vi "Power Output Unflatten Test Parameters.vi"(9 "error in (no error)":errorcluster, 10 "Parameter String":string) -> (1 "error out":errorcluster, 2 "Power Verification Test Parameters":T2={"Stimulus"={"Frequency Type"=enum."Band Edges", "Frequency Ranges"=[], "TX 1 Frequency (MHz)"={"Min"=0.0, "Max"=0.0}, "TX 2 Frequency (MHz)"={"Min"=0.0, "Max"=0.0}, "RX Frequency (MHz)"={"Min"=0.0, "Max"=0.0}, "Pad Model Number"="", "Pad Serial Number"="", "Pad Values"=[]}, "Measurement"={"DUT Port"=enum."Port 1", "Direction"=0, "Frequency Step Size"=0}, "Display"={"Frequency"={"Min"=-1.0, "Max"=-1.0}, "Power"={"Min"=-1, "Max"=-1}}, "Limit"={"Min Power (dBm)"=44.0}, "Calibration"={"Calibrated?"=FALSE}} {"Measurement"."Frequency Step Size" items=["0.2", "0.4", "1.0", "2.0", "4.0"]; "Measurement"."Direction" items=["Reverse", "Forward", "Auxiliary"]}, 5 "Test Version":string)   [LabVIEW 2011]
uses:
  TypeDefs/Power Output Test Parameters.ctl
  TypeDefs/Power Output Stimulus Parameters.ctl
  TypeDefs/Power Output Measurement Parameters.ctl
  SI.LIB/PIM.LIB/HW IO/DUTport.ctl
  SI.LIB/PIM.LIB/HW IO/MeasMode.ctl
  SI.LIB/PIM.LIB/HW IO/PIM Sweep Step Size.ctl
  TypeDefs/Power Output Display Parameters.ctl
  TypeDefs/Power Output Limit Parameters.ctl
  TypeDefs/Power Output Calibration State.ctl
  Test Return Parameter.ctl
panel:
  in  "Return Parameter":T1
  out "Parameter Variant":variant
  in  "Required Instruments":string[](array[string])=["PIM", "PWM"]
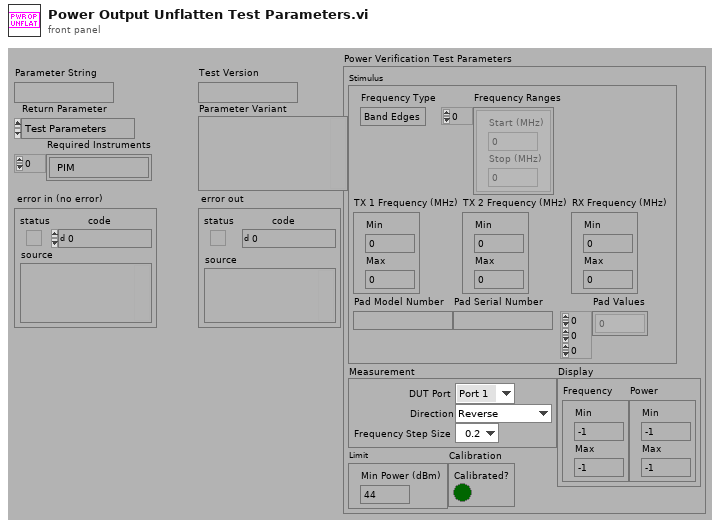
[diagram p1: front panel]
types:
  T1 = typedef "Test Return Parameter.ctl" = enum16{"Test Parameters", "Required Instruments", "Datasheets", "QuickMode"}
  T2 = typedef "Power Output Test Parameters.ctl" = cluster{"Stimulus":T3, "Measurement":T4, "Display":T8, "Limit":T9, "Calibration":T10}
  T3 = typedef "Power Output Stimulus Parameters.ctl" = cluster{"Frequency Type":enum16{"Band Edges", "Custom"}, "Frequency Ranges":cluster{"Start (MHz)":dbl, "Stop (MHz)":dbl}[], "TX 1 Frequency (MHz)":cluster{"Min":dbl, "Max":dbl}, "TX 2 Frequency (MHz)":cluster{"Min":dbl, "Max":dbl}, "RX Frequency (MHz)":cluster{"Min":dbl, "Max":dbl}, "Pad Model Number":string, "Pad Serial Number":string, "Pad Values":dbl[][][]}
  T4 = typedef "Power Output Measurement Parameters.ctl" = cluster{"DUT Port":T5, "Direction":T6, "Frequency Step Size":T7}
  T5 = typedef "DUTport.ctl" = enum16{"Port 1", "Port 2"}
  T6 = typedef "MeasMode.ctl" = u16
  T7 = typedef "PIM Sweep Step Size.ctl" = u16
  T8 = typedef "Power Output Display Parameters.ctl" = cluster{"Frequency":cluster{"Min":dbl, "Max":dbl}, "Power":cluster{"Min":i32, "Max":i32}}
  T9 = typedef "Power Output Limit Parameters.ctl" = cluster{"Min Power (dBm)":dbl}
  T10 = typedef "Power Output Calibration State.ctl" = cluster{"Calibrated?":bool}
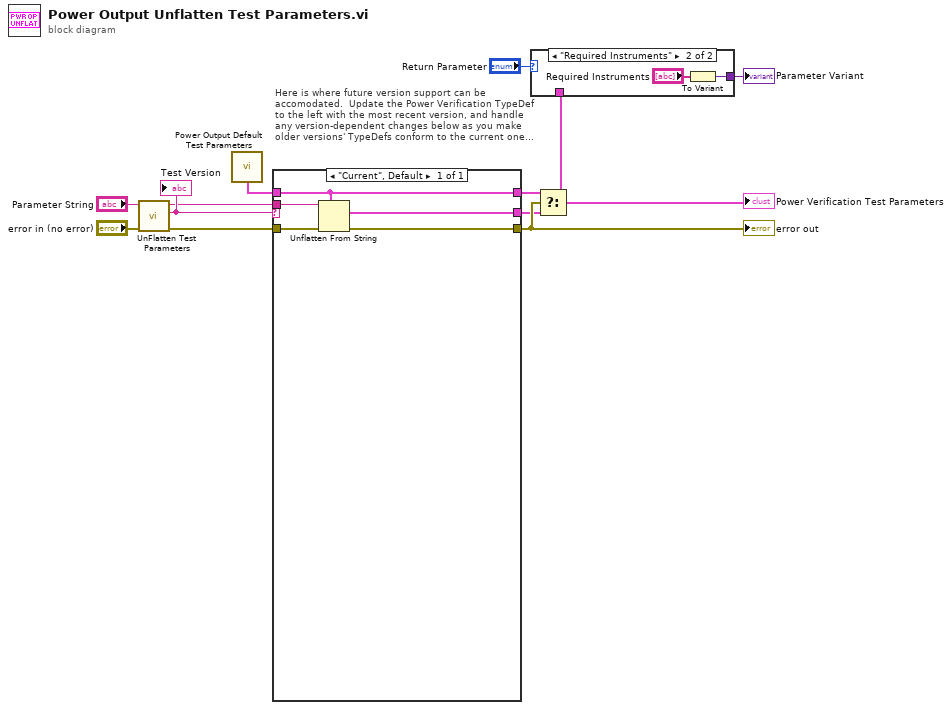
[diagram p0: block diagram]
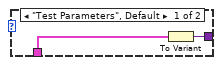
[diagram p2: hidden frame]
diagram:
  # "Here is where future version support can be\naccomodated.  Update the Power Verification TypeDef\nto the left with the most recent version, and handle\nany version-dependent changes below as you make\nolder versions' TypeDefs conform to the current one..."
  n1 = call "UnFlatten Test Parameters.vi"("error in (no error)"="error in (no error)", "Flattened Test Parameters with Version (\"\")"="Parameter String") -> ("error out"=w3:errorcluster, "Test Version"=w11:string, "Flat Test Parameters"=w10:string)  [unwired: 3 out]
  "Test Version" <- w11
  n2 = call "Power Output Default Test Parameters.vi"() -> ("Default Power Output Test Parameters"=w1:T2)
  n3 = case shown="\"Current\", Default" w11 {
    tunnel: w10 -> [w17]
    tunnel: w1 -> [w14]
    tunnel: [w16] -> w6
    tunnel: [w14] -> w9
    tunnel: w3 -> [w13]
    tunnel: [w15] -> w2
    frame "Current", Default {
      n4 = Unflatten From String(type=w14, binary string=w17, error in (no error)=w13) -> (value=w15:T2, error out=w16:errorcluster)  [unwired: 3 out]
    }
  }
  "error out" <- w6
  n5 = Select(t=w9, s=w6, f=w2) -> (s? t:f=w5:T2)
  "Power Verification Test Parameters" <- w5
  n6 = case shown="\"Required Instruments\"" "Return Parameter" {
    tunnel: [w19 w21] -> w7
    tunnel: w5 -> [w18 _]
    frame "Test Parameters", Default {
      n7 = To Variant(anything=w18) -> (Variant=w19:variant)
    }
    frame "Required Instruments" {
      n8 = To Variant(anything="Required Instruments") -> (Variant=w21:variant)
    }
  }
  "Parameter Variant" <- w7
